vi "Write MonoSettings.vi"(8 "error in (no error)":errorcluster, 10 "SetLimits":T1, 11 "Monochromator in":refnum<class "Monochromator.lvclass">) -> (0 "error out":errorcluster, 3 "Monochromator out":refnum<class "Monochromator.lvclass">)   [LabVIEW 2016, in "Monochromator.lvclass"]
uses:
  Monochromator.lvclass
  MonoSettings/Settings/ConfigurationTypedefs/Base/MonochromatorSettings.ctl
  Typedefs/wavelength.ctl
  Typedefs/slitWidth.ctl
  Monochromator.lvclass/Monochromator.ctl
  MonoSettings/Settings/ConfigurationTypedefs/ConfigurationTypedefs.lvlib
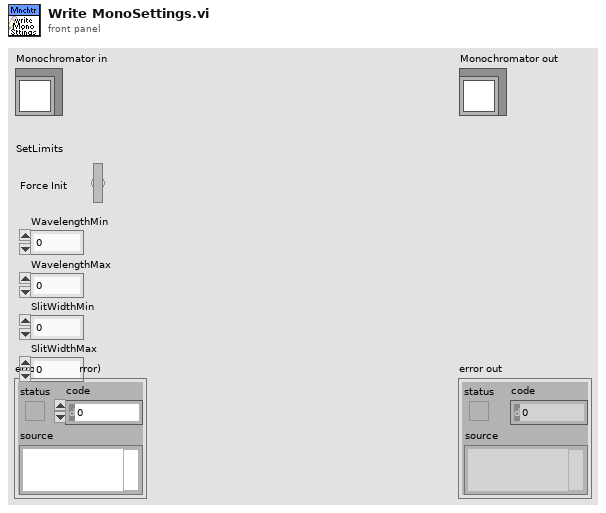
[diagram p1: front panel]
types:
  T1 = typedef "Settings.lvlib/ConfigurationTypedefs.lvlib/MonochromatorSettings.ctl" = cluster{"Force Init":bool, "WavelengthMin":T2, "WavelengthMax":T2, "SlitWidthMin":T3, "SlitWidthMax":T3}
  T2 = typedef "wavelength.ctl" = dbl
  T3 = typedef "slitWidth.ctl" = dbl
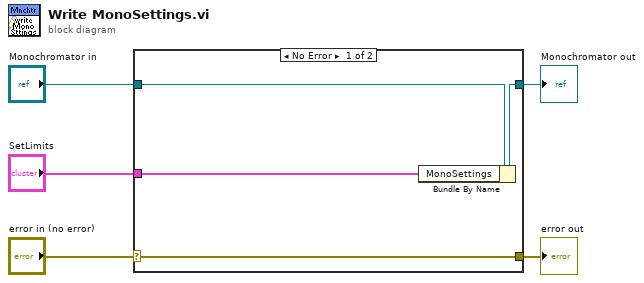
[diagram p0: block diagram]
diagram:
  n1 = case shown="No Error" "error in (no error)" {
    selector: "error in (no error)" -> [w9 w10]
    tunnel: [w9 w10] -> w4
    tunnel: [w7 w11] -> w2
    tunnel: "Monochromator in" -> [w8 w11]
    tunnel: "SetLimits" -> [w6 _]
    frame No Error {
      n2 = Bundle By Name(cluster=w8, "MonoSettings"=w6) -> (w7:refnum<class "Monochromator.lvclass">)
    }
    frame Error {
    }
  }
  "error out" <- w4
  "Monochromator out" <- w2
